vi "State_Machine.vi"(8 "error in (no error)":errorcluster caption="entrée d'erreur (pas d'erreur)", 11 "Delay en entrée":refnum<class "Reset_Variable_SIN.lvclass">) -> (0 "error out":errorcluster caption="sortie d'erreur", 2 "Json_String":string, 3 "Delay en sortie":refnum<class "Reset_Variable_SIN.lvclass">)   [LabVIEW 2020, in "Library Test.lvlib" / "Reset_Variable_SIN.lvclass"]
uses:
  Reset_Variable_SIN.lvclass
  Commun VI/TypeDef/Variable Printable.ctl
  Commun VI/Library Commun.lvlib
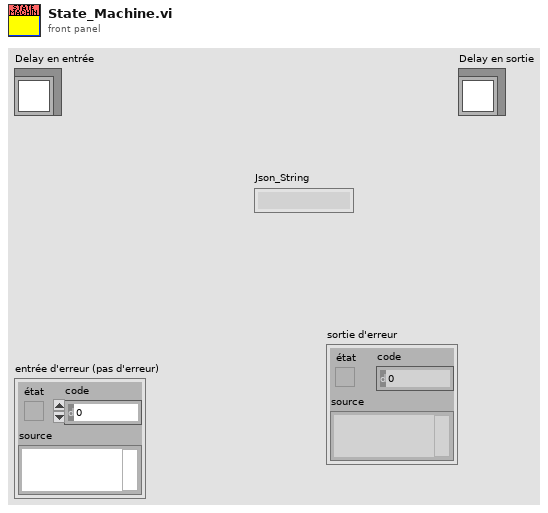
[diagram p1: front panel]
types:
  T1 = typedef "Variable Printable.ctl" = string
  T2 = enum16{"Get Variable", "Get All Variables", "Set Variable", "Delete Variable", "Delete All Variable"}
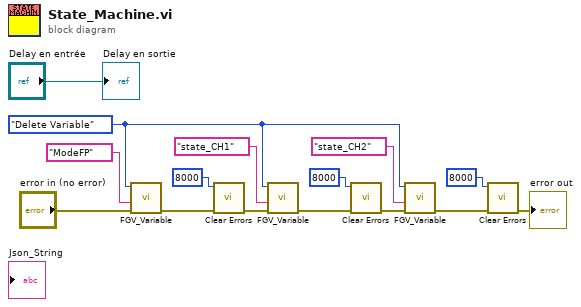
[diagram p0: block diagram]
diagram:
  w3 = T2."Delete Variable" ("Function")
  n1 = call "FGV_Variable.vi"("error in (no error)"="error in (no error)", "Variable"=T1 "ModeFP", "Function"=w3) -> ("error out"=w12:errorcluster)  [unwired: 6 in, 2 out]
  n2 = call <vilib>:"Clear Errors.vi"("error in (no error)"=w12, "specific error code to clear (0: all)"=8000) -> ("error out"=w11:errorcluster)  [unwired: 4 in, 1 out]
  n3 = call "FGV_Variable.vi"("error in (no error)"=w11, "Variable"=T1 "state_CH1", "Function"=w3) -> ("error out"=w2:errorcluster)  [unwired: 6 in, 2 out]
  n4 = call <vilib>:"Clear Errors.vi"("error in (no error)"=w2, "specific error code to clear (0: all)"=8000) -> ("error out"=w4:errorcluster)  [unwired: 4 in, 1 out]
  n5 = call "FGV_Variable.vi"("error in (no error)"=w4, "Variable"=T1 "state_CH2", "Function"=w3) -> ("error out"=w1:errorcluster)  [unwired: 6 in, 2 out]
  n6 = call <vilib>:"Clear Errors.vi"("error in (no error)"=w1, "specific error code to clear (0: all)"=8000) -> ("error out"=→"error out":errorcluster)  [unwired: 4 in, 1 out]
  "Delay en sortie" <- "Delay en entrée"
